vi "water-tank.vi"() -> ()   [LabVIEW 2019]
panel:
  out "Alarm":bool
  out "Rain":bool
  in  "Irrigation OFF (Automatic mode)":dbl
  in  "Irrigation ON (Automatic mode)":dbl
  in  "Irrigation (Manual mode)":bool
  out "Days":dbl
  out "Clock":dbl(knob) scale=0.0..24.0
  out "Filling":bool
  in  "stop":bool
  in  "Automatic/Manual":bool
  out "Maximum":bool
  out "Minimum":bool
  in  "Filling the tank\nON/OFF":bool
  out "Tank":dbl(slide) scale=0.0..100.0
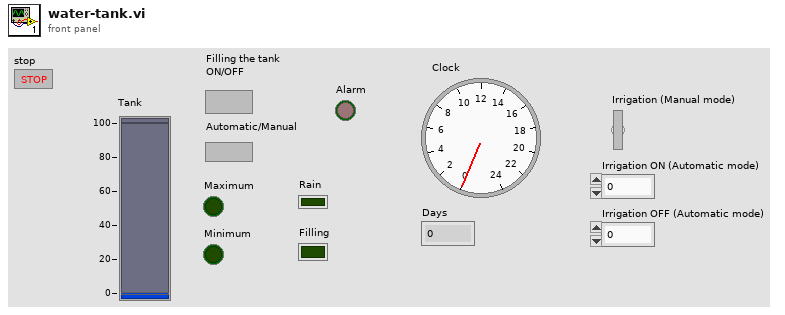
[diagram p1: front panel]
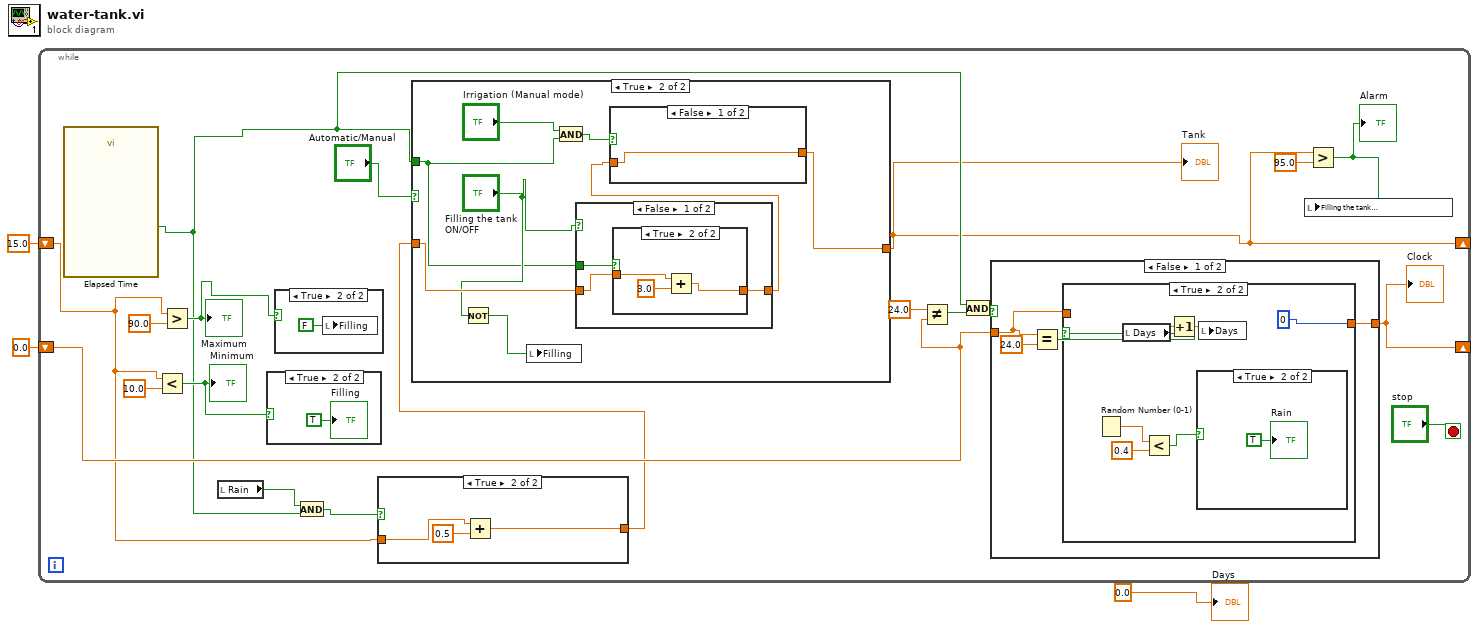
[diagram p0: block diagram]
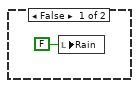
[diagram p4: hidden frame]
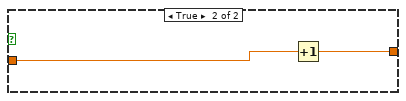
[diagram p5: hidden frame]
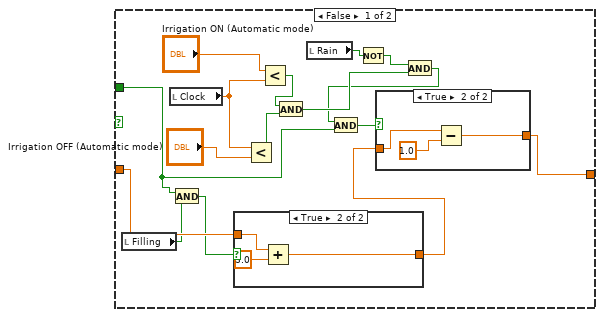
[diagram p8: hidden frame]
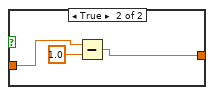
[diagram p11: hidden frame]
diagram:
  n1 = while {
    shift-right: [w6] -> _
    shift-left: 15.0 -> [w8]
    shift-right: [w16] -> _
    shift-left: 0.0 -> [w13]
    stop <- "stop" stop-if-true
    n2 = call "Elapsed Time"() -> ("Time has Elapsed"=w10:bool)  [unwired: 12 in, 7 out]
    n3 = Less?(x=w8, y=10.0) -> (x < y?=w18:bool)
    "Minimum" <- w18
    n4 = Greater?(x=w8, y=90.0) -> (0:w17:bool)
    "Maximum" <- w17
    n5 = local read "Rain"() -> (w11:bool)
    n6 = case shown="True" w18 {
      frame False {
      }
      frame True {
        "Filling" <- TRUE ("Filling")
      }
    }
    n7 = case shown="True" w17 {
      frame False {
      }
      frame True {
        n8 = local write "Filling"(FALSE ("Filling")) -> ()
      }
    }
    n9 = And(x=w11, y=w10) -> (x .and. y?=w9:bool)
    n10 = case shown="True" w9 {
      tunnel: w8 -> [w23 w25]
      tunnel: [w23 w24] -> w7
      frame False {
      }
      frame True {
        n11 = Add(x=w25, y=0.5) -> (x+y=w24:dbl)
      }
    }
    n12 = case shown="True" "Automatic/Manual" {
      tunnel: w7 -> [w59 w75]
      tunnel: [w56 w71] -> w6
      tunnel: w10 -> [w48 w68]
      frame False {
        n13 = local read "Filling"() -> (w57:bool)
        n14 = local read "Clock"() -> (w53:dbl)
        n15 = And(x=w48, y=w57) -> (x .and. y?=w58:bool)
        n16 = case shown="True" w58 {
          tunnel: w59 -> [w64 w66]
          tunnel: [w64 w65] -> w55
          frame False {
          }
          frame True {
            n17 = Add(x=w66, y=3.0) -> (x+y=w65:dbl)
          }
        }
        n18 = Less?(x=w53, y="Irrigation OFF (Automatic mode)") -> (x < y?=w50:bool)
        n19 = Less?(x="Irrigation ON (Automatic mode)", y=w53) -> (x < y?=w51:bool)
        n20 = And(x=w51, y=w50) -> (x .and. y?=w45:bool)
        n21 = local read "Rain"() -> (w47:bool)
        n22 = Not(x=w47) -> (.not. x?=w46:bool)
        n23 = And(x=w46, y=w45) -> (x .and. y?=w44:bool)
        n24 = And(x=w44, y=w48) -> (x .and. y?=w49:bool)
        n25 = case shown="True" w49 {
          tunnel: [w60 w62] -> w56
          tunnel: w55 -> [w60 w61]
          frame False {
          }
          frame True {
            n26 = Subtract(x=w61, y=1.0) -> (x-y=w62:dbl)
          }
        }
      }
      frame True {
        n27 = Not(x="Filling the tank\nON/OFF") -> (.not. x?=w74:bool)
        n28 = local write "Filling"(w74) -> ()
        n29 = And(x="Irrigation (Manual mode)", y=w68) -> (x .and. y?=w69:bool)
        n30 = case shown="False" "Filling the tank\nON/OFF" {
          tunnel: w75 -> [w82 w87]
          tunnel: [w81 w87] -> w72
          tunnel: w68 -> [w80 _]
          frame False {
            n31 = case shown="True" w80 {
              tunnel: w82 -> [w83 w85]
              tunnel: [w83 w86] -> w81
              frame False {
              }
              frame True {
                n32 = Add(x=w85, y=3.0) -> (x+y=w86:dbl)
              }
            }
          }
          frame True {
          }
        }
        n33 = case shown="False" w69 {
          tunnel: w72 -> [w76 w78]
          tunnel: [w76 w77] -> w71
          frame False {
          }
          frame True {
            n34 = Subtract(x=w78, y=1.0) -> (x-y=w77:dbl)
          }
        }
      }
    }
    "Tank" <- w6
    n35 = Not Equal?(x=24.0, y=w13) -> (x != y?=w14:bool)
    n36 = And(x=w10, y=w14) -> (x .and. y?=w15:bool)
    n37 = case shown="False" w15 {
      tunnel: [w28 w41] -> w16
      tunnel: w13 -> [w27 w40]
      frame False {
        n38 = Equal?(x=w27, y=24.0) -> (x = y?=w29:bool)
        n39 = case shown="True" w29 {
          tunnel: [w31 0] -> w28
          tunnel: w27 -> [w31 _]
          frame False {
          }
          frame True {
            n40 = Random Number (0-1)() -> (number: 0 to 1=w34:dbl)
            n41 = local read "Days"() -> (w35:dbl)
            n42 = Less?(x=w34, y=0.4) -> (x < y?=w32:bool)
            n43 = Increment(x=w35) -> (x+1=w36:dbl)
            n44 = case shown="True" w32 {
              frame False {
                n45 = local write "Rain"(FALSE ("Rain")) -> ()
              }
              frame True {
                "Rain" <- TRUE ("Rain")
              }
            }
            n46 = local write "Days"(w36) -> ()
          }
        }
      }
      frame True {
        n47 = Increment(x=w40) -> (x+1=w41:dbl)
      }
    }
    "Clock" <- w16
    n48 = Greater?(x=w6, y=95.0) -> (0:w4:bool)
    "Alarm" <- w4
    n49 = local write "Filling the tank\nON/OFF"(w4) -> ()
  }
  "Days" <- 0.0 ("Days")
